vi "VI Property Node.vi"   [LabVIEW 2017]
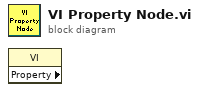
[diagram p0: block diagram]
diagram:
  n1 = property class="VI" props=[]() -> ()  [unwired: 2 in, 3 out]
